vi "APS arc2 ca v.vi"(0 "Axis_ID_Array":i32, 1 "TransPara":dbl, 2 "Wait":cluster{"h_event":u32, "i32_ret":i32}, 5 "Option":i32, 7 "CenterArray":dbl, 9 "Angle":dbl, 11 "error in (no error)":errorcluster caption="错误输入（无错误）", 12 "Vm":dbl) -> (3 "TransPara out":dbl, 4 "Axis_ID_Array out":i32, 6 "Wait out":cluster{"h_event":u32, "i32_ret":i32}, 8 "CenterArray out":dbl, 10 "function return":i32, 15 "error out":errorcluster caption="错误输出")   [LabVIEW 2017, in "APS168.lvlib"]
doc: "I32 FNTYPE APS_arc2_ca_v( I32 *Axis_ID_Array, I32 Option, F64 *CenterArray, F64 Angle, F64 *TransPara, F64 Vm, ASYNCALL *Wait );"
uses:
  APS168.lvlib
  APS168.dll
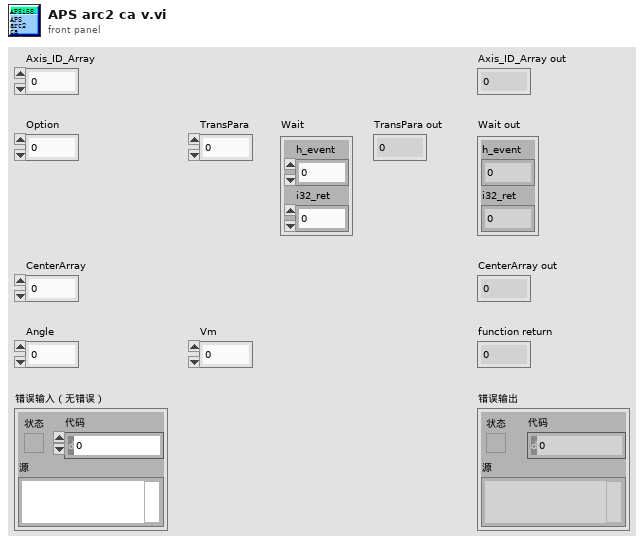
[diagram p1: front panel]
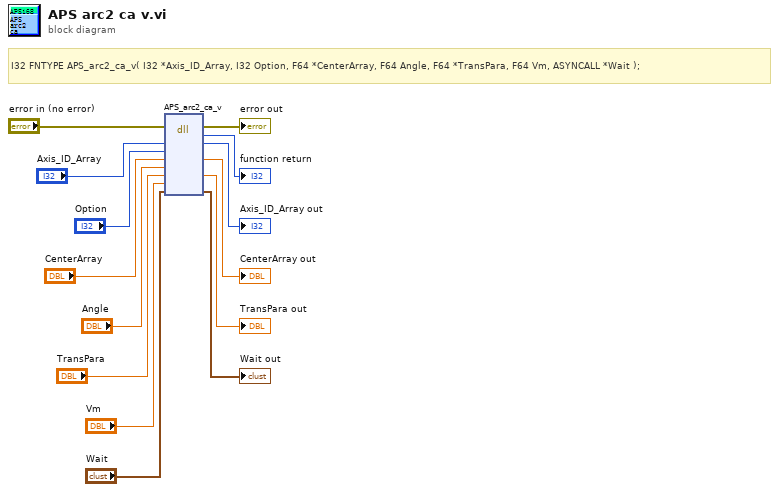
[diagram p0: block diagram]
diagram:
  # "I32 FNTYPE APS_arc2_ca_v( I32 *Axis_ID_Array, I32 Option, F64 *CenterArray, F64 Angle, F64 *TransPara, F64 Vm, ASYNCALL *Wait );"
  n1 = dll-call lib="PTH2Gabs E迈治LV范例testSubVIsADLINKMotion204cAPS168.*" fn="APS_arc2_ca_v"(error in="error in (no error)", "Axis_ID_Array"="Axis_ID_Array", "Option"="Option", "CenterArray"="CenterArray", "Angle"="Angle", "TransPara"="TransPara", "Vm"="Vm", "Wait"="Wait") -> (error out=→"error out":errorcluster, →"function return":i32, "Axis_ID_Array"=→"Axis_ID_Array out":i32, "CenterArray"=→"CenterArray out":dbl, "TransPara"=→"TransPara out":dbl, "Wait"=→"Wait out":cluster{"h_event":u32, "i32_ret":i32})  [unwired: 5 in, 1 out]
